vi "Set Window State.vi"(6 "State":T1(ring), 8 "error in (no error)":errorcluster, 11 "Actor API in":refnum<class "Actor API.lvclass">) -> (0 "error out":errorcluster)   [LabVIEW 2020, in "Actor API.lvclass"]
uses:
  Actor API.lvclass
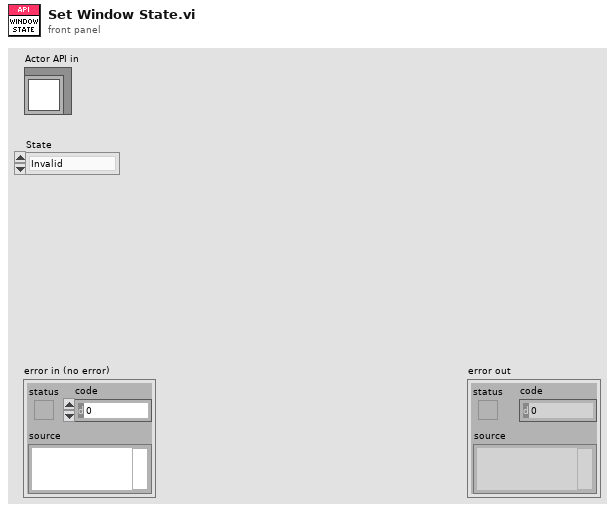
[diagram p1: front panel]
types:
  T1 = enum32{"Invalid", "Standard", "Closed", "Hidden", "Minimized", "Maximized"}
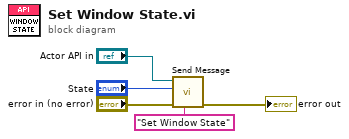
[diagram p0: block diagram]
diagram:
  n1 = call "Send Message.vi"("Name"="Set Window State", "error in (no error)"="error in (no error)", "Payload"="State", "Actor API in"="Actor API in") -> ("error out"=→"error out":errorcluster)  [unwired: 7 in]
